vi "HOST_phasedelaycheck_11-19.vi"() -> ()   [LabVIEW 2020]
uses:
  <vilib>/userDefined/Silver/nirio_resource_slv.ctl
  Controls/Clock Select.ctl
  <vilib>/FPGAPlugInAG/PXIe-7972R/niLvFpga_Open_PXIe-7972R.vi
  <vilib>/rvi/interface/common/dynamic/niFpgaDynamicAddResources.vi
  <vilib>/rvi/interface/common/niFpgaWaitOnOcc.vi
  <vilib>/Utility/error.llb/Error Cluster From Error Code.vi
  <vilib>/rvi/errors/niLvFpgaAdjustHostInterfaceError.vi
  <instrlib>/_niInstr/Streaming/v1/Host/Public/Start Finite Stream.vi
  <instrlib>/_niInstr/Streaming/v1/Host/Public/Wait for Stream.vi
  <instrlib>/_niInstr/Streaming/v1/Host/Public/Start Continuous Stream.vi
  <vilib>/FPGAPlugInAG/Dynamic/niLvFpga_Close_Dynamic.vi
  <vilib>/rvi/interface/nirviOpenFPGA/nirviOpenFPGA.xnode
  FPGA Bitfiles/rfsignal_FPGATarget_phasedelaycheck1_neufEMLyap0.lvbitx
  <vilib>/rvi/interface/nirviMethod/nirviMethod.xnode
  <vilib>/rvi/interface/nirviReadWriteControl/nirviReadWriteControl.xnode
  <vilib>/rvi/interface/nirviCloseFPGA/nirviCloseFPGA.xnode
  <vilib>/rvi/errors/niLvFpgaMergeErrorWithErrorCode.vi
  <instrlib>/_niInstr/Streaming/v1/Host/niInstr Streaming v1 Host.lvlib
  <vilib>/rvi/interface/Simulation/niFpgaSimulationCallBeginRW.vi
  NiFpgaLv.dll
  <vilib>/FPGAPlugInAG/Dynamic/niLvFpga_ConfigureFifo_Dynamic.vi
  <vilib>/FPGAPlugInAG/Dynamic/niLvFpga_StartFifo_Dynamic.vi
  <vilib>/FPGAPlugInAG/Dynamic/niLvFpga_WriteFifo_Dynamic.vi
panel:
  in  "Testing setting":T1(ring)
  in  "CH0 Amp inc/dec":u8[](array[ring])=[0, 0, 0, 0, 0, 0, 0, 0, 0, 0] items=["", "Increase", "Decrease"]
  in  "CH0 Freq inc/dec":u8[](array[ring])=[0, 0, 0, 0, 0, 0, 0, 0, 0, 0] items=["", "Increase", "Decrease"]
  in  "CH1 Amp inc/dec":u8[](array[ring])=[0, 0, 0, 0, 0, 0, 0, 0, 0, 0] items=["", "Increase", "Decrease"]
  in  "CH1 Freq inc/dec":u8[](array[ring])=[0, 0, 0, 0, 0, 0, 0, 0, 0, 0] items=["", "Increase", "Decrease"]
  out "AI 2 beam 1":cluster{"AI0":i16, "AI3":i16}(graph)={"AI0"=37, "AI3"=37}
  out "AI 1 beam 1":cluster{"AI0":i16, "AI3":i16}(graph)={"AI0"=-70, "AI3"=-70}
  out "AI 0 beam 1":cluster{"AI0":i16, "AI3":i16}(graph)={"AI0"=-27, "AI3"=-27}
  in  "Norm % 2":dbl=1.0 format="%#_13g"
  in  "Norm %":dbl=1.0 format="%#_13g"
  in  "Gain X %/s":fxp<+/-,64,32>
  in  "Gain Y %/s":fxp<+/-,64,32>
  in  "X (CH1) Hz/s":fxp<+/-,64,32>
  in  "Y (CH0) Hz/s":fxp<+/-,64,32>
  in  "Input pass through\nmode":enum16{"Wire", "Accum", "Accum-edge"}(ring)
  in  "# of beams":i8=1
  in  "Wave Reader CH 1 (X)":fxp<+/-,64,32>[](array[numeric])=[27000000.0, 26000000.0, 28000000.0, 25000000.0, 21000000.0, 25000000.0, 30000000.0, 34000000.0, 27000000.0] format="%_17p"
  in  "Gain CH 1 (multiplicative)":fxp<+,32,4>[](array[numeric])=[1.0, 1.0, 0.9999999925494194, 1.0, 1.0, 1.0, 1.0, 1.0, 1.0]
  in  "Remove transition edges":i32=5
  in  "Time per beam in us":i32=20
  in  "stop":bool
  in  "Gain CH 0 (multiplicative)":fxp<+,32,4>[](array[numeric])=[1.0, 1.0, 1.0, 1.0, 1.0, 1.0, 1.0, 1.0, 1.0]
  in  "Wave Reader CH 0 (Y)":fxp<+/-,64,32>[](array[numeric])=[27000000.0, 26000000.0, 28000000.0, 25000000.0, 21000000.0, 25000000.0, 30000000.0, 34000000.0, 27000000.0] format="%_17p"
  out "AO":waveform(dbl)(graph)={"t0"=timestamp(0.0004 s since 1904-01-01), "dt"=6.103515625e-09, "Y"=array[65536 elements]}
  in  "Magnitude Initialization Vpp":dbl[](array[numeric])=[1.0, 1.0] format="%0.2p"
  in  "Frequencies (Hz)":dbl[](array[numeric])=[10000.0, 10000.0] format="%5.0p"
  in  "Signal Type":T2(ring)
  in  "Sampling Info":cluster{"Fs":dbl, "#s":dbl}={"Fs"=163840000.0, "#s"=65536.0} {"Fs" format="%#_5p"}
  out "Error Out":errorcluster
  in  "Update Waveform":bool
  in  "Clock Select":T3 items=["Internal Clock", "Internal Clock w/ Ref via CLK/REF IN", "Internal Clock w/ Ref via Sync Clock", "External Clock via CLK/REF IN"]
  in  "Rate of External Sample Clock (MHz)":u16=100 min=60 max=100 step=1
  in  "RIO Resource":T4="PXI1Slot5"
  # "General Feedback Settings"
  # "Time cycle loop processing"
  # "Shared Feedback Controls"
  # "Don't change"
  # "Waveform Initialization"
  # "DO NOT CHANGE"
  # "Ch 0 Output Waveforms"
  # "Ch 1 Output Waveforms"
  # "Initialization waveform stored in FPGA"
  # "Ch0"
  # "Ch1"
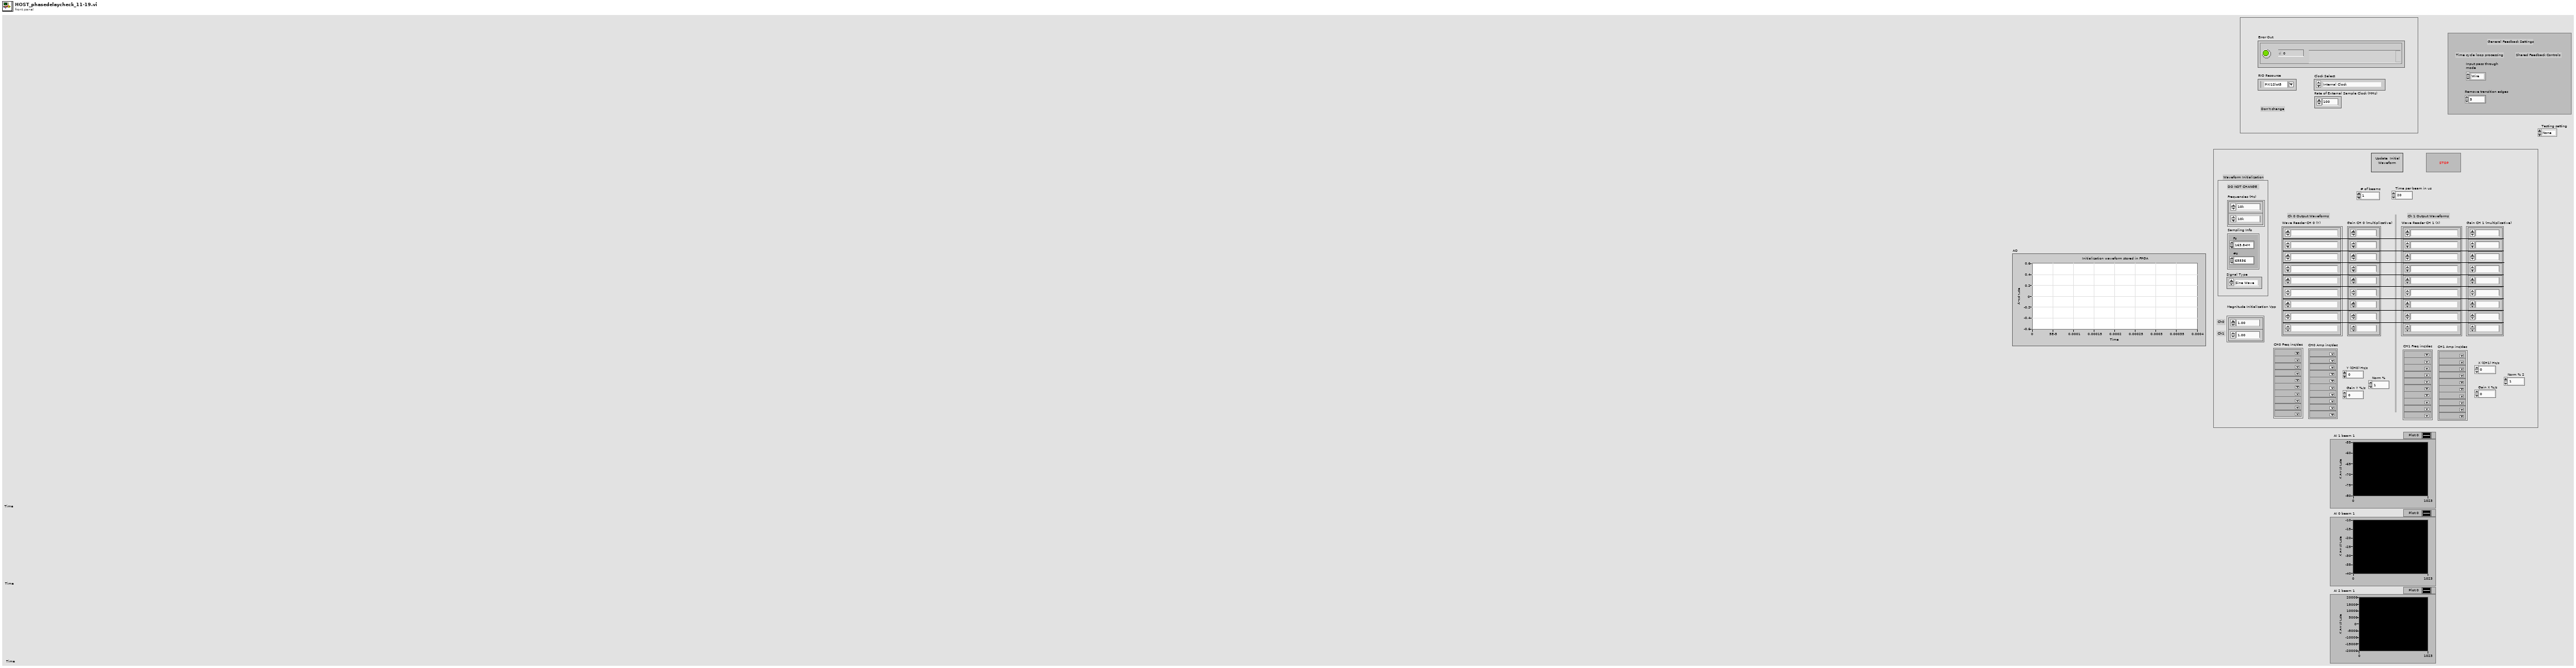
[diagram p1: front panel]
types:
  T1 = enum16{"None", "AI", "Y and Z", "X and Z", "input loop"}
  T2 = enum16{"Sine Wave", "Triangle Wave", "Square Wave", "Sawtooth Wave"}
  T3 = typedef "Clock Select.ctl" = u16
  T4 = typedef "nirio_resource_slv.ctl" = tag
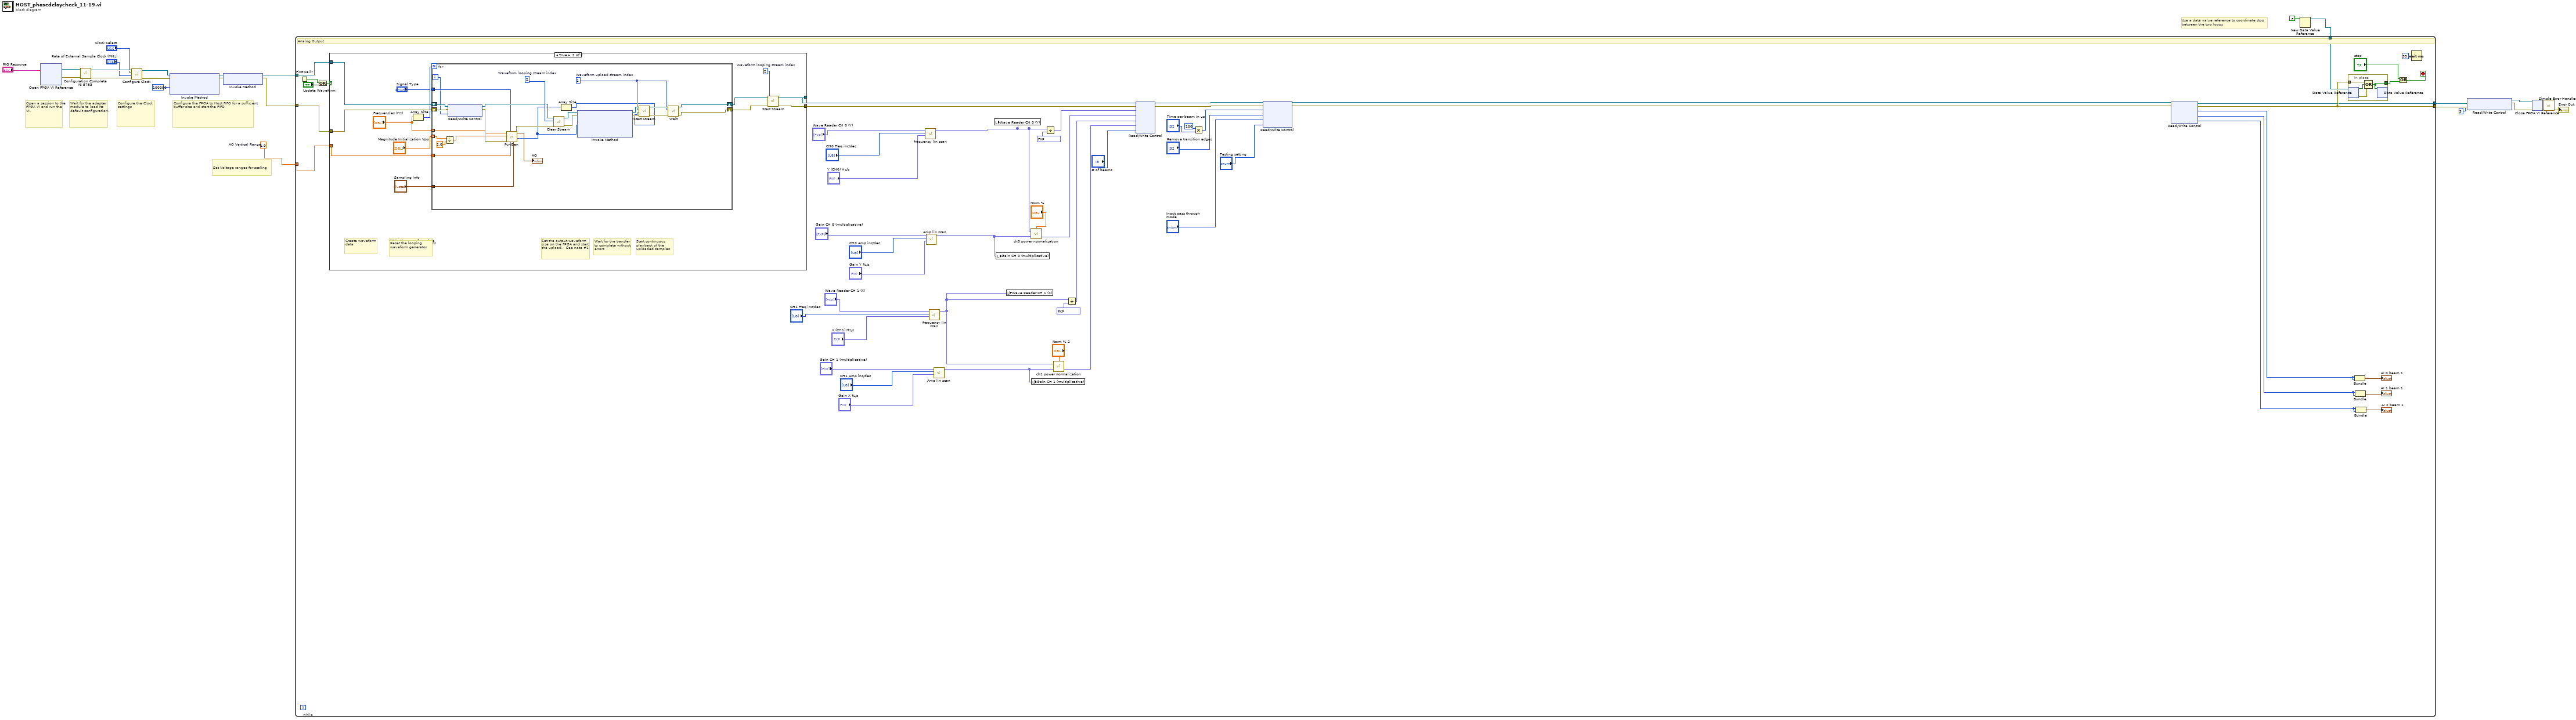
[diagram p0: block diagram]
diagram:
  w12 = 1.0  # AO Vertical Range
  # "Use a data value reference to coordinate stop between the two loops"
  # "Set Voltage ranges for scaling"
  # "Configure the Clock settings"
  # "Configure the FPGA to Host FIFO for a sufficient buffer size and start the FIFO"
  # "Wait for the adapter module to load its default configuration."
  # "Open a session to the FPGA VI and run the VI."
  n1 = xnode "Open FPGA VI Reference"("resource name"="RIO Resource") -> ("FPGA VI Reference Out"=w10:refnum<k20>, "error out"=w9:errorcluster)  [unwired: 1 in]
  n2 = call "Configuration Complete NI 5783.vi"("error in"=w9, "FPGA VI Reference In"=w10) -> ("error out"=w20:errorcluster, "FPGA VI Reference Out"=w21:refnum<k20>)  [unwired: 7 in, 1 out]
  n3 = call "Configure Clock.vi"("error in (no error)"=w20, "Rate of External Sample Clock (MHz)"="Rate of External Sample Clock (MHz)", "Clock Select"="Clock Select", "FPGA VI Reference In"=w21) -> ("error out"=w18:errorcluster, "FPGA VI Reference Out"=w19:refnum<k20>)  [unwired: 3 in, 3 out]
  n4 = xnode "Invoke Method"("FPGA VI Reference In"=w19, "error in"=w18, "Requested Depth"=u32 100000) -> ("FPGA VI Reference Out"=w24:refnum<k20>, "error out"=w23:errorcluster)  [unwired: 1 out]
  n5 = xnode "Invoke Method"("FPGA VI Reference In"=w24, "error in"=w23) -> ("FPGA VI Reference Out"=w3:refnum<k20>, "error out"=w2:errorcluster)
  n6 = New Data Value Reference(data value=FALSE ("Stopped")) -> (data value reference=w1:refnum<data-value>)  [unwired: 1 in, 1 out]
  n7 = while {
    tunnel: w2 -> [w74]
    tunnel: [w43] -> w8
    tunnel: w3 -> [w80]
    tunnel: [w36] -> w7
    tunnel: w1 -> [w75]
    tunnel: w12 -> [w73]
    stop <- w70 stop-if-true
    # "Analog Output"
    n8 = First Call?() -> (First Call?: T/F=w76:bool)
    n9 = Or(x=w76, y="Update Waveform") -> (x .or. y?=w77:bool)
    n10 = case shown="True" w77 {
      tunnel: [w86 w99] -> w72
      tunnel: [w85 w98] -> w71
      tunnel: w80 -> [w86 w96]
      tunnel: w74 -> [w85 w95]
      tunnel: w73 -> [_ w97]
      frame False {
      }
      frame True {
        w94 = 2  # Waveform looping stream index
        # "Loop over the waveforms to combine"
        # "Reset the looping waveform generator"
        # "Start continuous playback of the uploaded samples"
        # "Wait for the transfer to complete without errors"
        # "Set the output waveform size on the FPGA and start the upload.   See note #1"
        # "Write the waveform data to the FPGA for generation"
        # "Create waveform data"
        n11 = Array Size(array="Frequencies (Hz)") -> (size(s)=w89:i32)
        n12 = for {
          N: w89 -> [_]
          tunnel: w97 -> [w115]
          shift-right: [w109] -> w93
          shift-left: w96 -> [w114]
          shift-right: [w108] -> w92
          shift-left: w95 -> [w112]
          tunnel: "Frequencies (Hz)" -> [w107] mode=indexing
          tunnel: "Magnitude Initialization Vpp" -> [w103] mode=indexing
          tunnel: "Sampling Info" -> [w106]
          tunnel: "Signal Type" -> [w105]
          i -> [w104]
          w116 = 2  # Waveform looping stream index
          w121 = 1  # Waveform upload stream index
          n13 = Divide(x=w103, y=2.0) -> (x/y=w102:dbl)
          n14 = xnode "Read/Write Control"("FPGA VI Reference In"=w114, "error in"=w112, "Upload selector"=w104) -> ("FPGA VI Reference Out"=w113:refnum<k20>, "error out"=w111:errorcluster)
          n15 = call "FunGen.vi"("sampling info"=w106, "range (Vpp)"=w115, "signal type"=w105, "error in (no error)"=w111, "amplitude"=w102, "frequency"=w107) -> ("error out"=w117:errorcluster, "Waveform Data"=w110:i16[], "Output Waveform (V)"=→"AO":waveform(dbl))  [unwired: 2 in, 1 out]
          n16 = call <instrlib>:"Clear Stream.vi"("error in (no error)"=w117, "stream index"=w116, "refnum in"=w113) -> ("error out"=w119:errorcluster, "refnum out"=w120:refnum<k20>)  [unwired: 7 in]
          n17 = Array Size(array=w110) -> (size(s)=w118:i32)
          n18 = xnode "Invoke Method"("FPGA VI Reference In"=w120, "error in"=w119, "Data"=w110) -> ("FPGA VI Reference Out"=w125:refnum<k20>, "error out"=w124:errorcluster)  [unwired: 1 in, 1 out]
          n19 = call-poly <instrlib>:"Start Stream.vi"("error in (no error)"=w124, "num samples"=w118, "stream index"=w121, "refnum in"=w125) -> ("error out"=w122:errorcluster, "refnum out"=w123:refnum<k20>)  [unwired: 6 in]
          n20 = call-poly <instrlib>:"Wait.vi"("error in (no error)"=w122, "stream index"=w121, "refnum in"=w123) -> ("error out"=w108:errorcluster, "refnum out"=w109:refnum<k20>)  [unwired: 5 in, 2 out]
        }
        n21 = call-poly <instrlib>:"Start Stream.vi"("error in (no error)"=w92, "stream index"=w94, "refnum in"=w93) -> ("error out"=w98:errorcluster, "refnum out"=w99:refnum<k20>)  [unwired: 7 in]
      }
    }
    n22 = call "frequency lin scan.vi"("Hz/s"="Y (CH0) Hz/s", "Freq inc/dec"="CH0 Freq inc/dec", "Wave Reader"="Wave Reader CH 0 (Y)") -> ("Array"=w34:fxp<+/-,64,32>[])  [unwired: 8 in]
    n23 = call "Amp lin scan.vi"("Gain %/s"="Gain Y %/s", "Amp inc/dec"="CH0 Amp inc/dec", "Gain"="Gain CH 0 (multiplicative)") -> ("Array"=w29:fxp<+,32,4>[])  [unwired: 8 in]
    n24 = call "frequency lin scan.vi"("Hz/s"="X (CH1) Hz/s", "Freq inc/dec"="CH1 Freq inc/dec", "Wave Reader"="Wave Reader CH 1 (X)") -> ("Array"=w47:fxp<+/-,64,32>[])  [unwired: 8 in]
    n25 = call "Amp lin scan.vi"("Gain %/s"="Gain X %/s", "Amp inc/dec"="CH1 Amp inc/dec", "Gain"="Gain CH 1 (multiplicative)") -> ("Array"=w49:fxp<+,32,4>[])  [unwired: 8 in]
    n26 = local write "Wave Reader CH 0 (Y)"(w34) -> ()
    n27 = local write "Gain CH 0 (multiplicative)"(w29) -> ()
    n28 = local write "Wave Reader CH 1 (X)"(w47) -> ()
    n29 = call "ch0 power normalization.vi"("% of max"="Norm %", "Gain"=w29, "Wave freq"=w34) -> ("Array"=w45:fxp<+,32,2>[])
    n30 = local write "Gain CH 1 (multiplicative)"(w49) -> ()
    n31 = Divide(x=w34, y=fxp<+,32,16> 6103.515625) -> (x/y=w61:fxp<+,32,16>[])
    n32 = call "ch1 power normalization.vi"("% of max"="Norm % 2", "Gain"=w49, "Wave freq"=w47) -> ("Array"=w48:fxp<+,32,2>[])
    n33 = Divide(x=w47, y=fxp<+,32,16> 6103.515625) -> (x/y=w59:fxp<+,32,16>[])
    n34 = xnode "Read/Write Control"("FPGA VI Reference In"=w72, "error in"=w71, "Wave 1"=w61, "Amp 1"=w45, "Wave 2"=w59, "Amp 2"=w48, "Size"="# of beams") -> ("FPGA VI Reference Out"=w66:refnum<k20>, "error out"=w65:errorcluster)
    n35 = Multiply(x=100, y="Time per beam in us") -> (x*y=w62:i32)
    n36 = xnode "Read/Write Control"("FPGA VI Reference In"=w66, "error in"=w65, "Timeshare"=w62, "Edge size"="Remove transition edges", "Pass selector"="Input pass through\nmode", "Test setting"="Testing setting") -> ("FPGA VI Reference Out"=w51:refnum<k20>, "error out"=w50:errorcluster)
    n37 = xnode "Read/Write Control"("FPGA VI Reference In"=w51, "error in"=w50) -> ("FPGA VI Reference Out"=w36:refnum<k20>, "error out"=w43:errorcluster, "AI 0 input 1"=w39:i16, "AI 1 input 1"=w38:i16, "AI 2 input 1"=w37:i16)
    n38 = in-place {
      in-place-border: [w82] -> w69
      in-place-border: w43 -> [w84]
      n39 = in-place-dvr #1(w75) -> (w83:bool, w81:errorcluster)
      n40 = Compound Arithmetic op=OR(w84, w83, w81) -> (w82:bool)
      n41 = in-place-dvr #1(w82) -> ()  [unwired: 2 out]
    }
    n42 = Bundle("AI 0 input 1"=w39, "AI 0 input 1"=w39) -> (→"AI 0 beam 1":cluster{"AI 0 input 1":i16, "AI 0 input 1":i16})  [unwired: 1 in]
    n43 = Bundle("AI 1 input 1"=w38, "AI 1 input 1"=w38) -> (→"AI 1 beam 1":cluster{"AI 1 input 1":i16, "AI 1 input 1":i16})  [unwired: 1 in]
    n44 = Bundle("AI 2 input 1"=w37, "AI 2 input 1"=w37) -> (→"AI 2 beam 1":cluster{"AI 2 input 1":i16, "AI 2 input 1":i16})  [unwired: 1 in]
    n45 = Or(x="stop", y=w69) -> (x .or. y?=w70:bool)
    n46 = Wait (ms)(milliseconds to wait=u32 33) -> ()  [unwired: 1 out]
  }
  n47 = xnode "Read/Write Control"("FPGA VI Reference In"=w7, "error in"=w8, "stream.request state 2"=3) -> ("FPGA VI Reference Out"=w4:refnum<k20>, "error out"=w6:errorcluster)
  n48 = xnode "Close FPGA VI Reference"("FPGA VI Reference In"=w4, "error in"=w6) -> ("error out"=w15:errorcluster)
  n49 = call <vilib>:"Simple Error Handler.vi"("error in (no error)"=w15) -> ("error out"=→"Error Out":errorcluster)  [unwired: 4 in, 4 out]
